vi "Write Master Motor Controller Config.vi"(8 "error in (no error)":errorcluster, 10 "Master Motor Controller Config":T1, 11 "Comp Motors with Encoders in":refnum<class "Comp Motors with Encoders.lvclass">) -> (0 "error out":errorcluster, 3 "Comp Motors with Encoders out":refnum<class "Comp Motors with Encoders.lvclass">)   [LabVIEW 2014, in "Comp Motors with Encoders.lvlib" / "Comp Motors with Encoders.lvclass"]
uses:
  Comp Motors with Encoders.lvclass
  Motor Controller Config.ctl
  Comp Motors with Encoders.lvclass/Comp Motors with Encoders.ctl
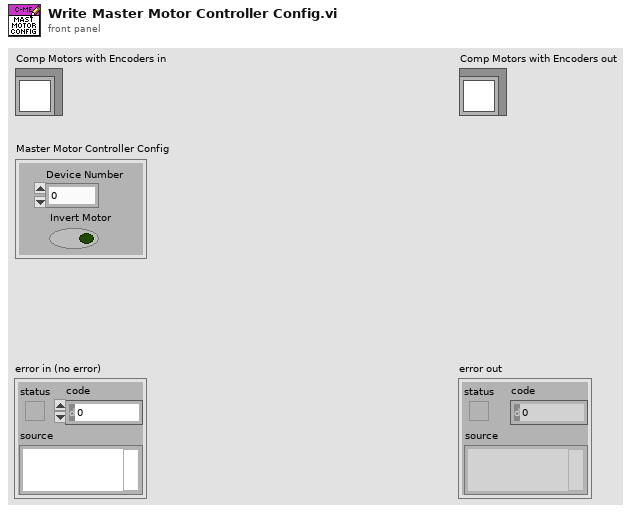
[diagram p1: front panel]
types:
  T1 = typedef "Comp Motors with Encoders.lvlib/Comp Motors with Encoders.lvclass/Motor Controller Config.ctl" = cluster{"Device Number":u8, "Invert Motor":bool}
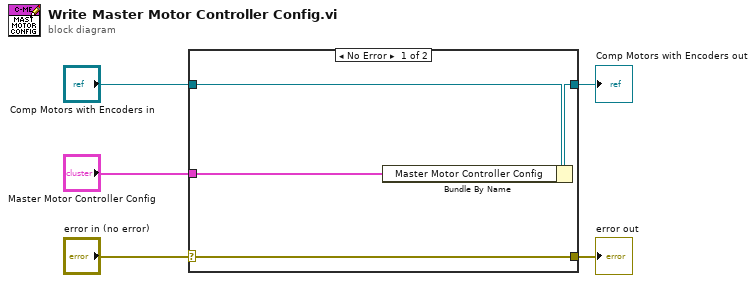
[diagram p0: block diagram]
diagram:
  n1 = case shown="No Error" "error in (no error)" {
    selector: "error in (no error)" -> [w9 w10]
    tunnel: [w9 w10] -> w4
    tunnel: [w7 w11] -> w2
    tunnel: "Comp Motors with Encoders in" -> [w8 w11]
    tunnel: "Master Motor Controller Config" -> [w6 _]
    frame No Error {
      n2 = Bundle By Name(cluster=w8, "Master Motor Controller Config"=w6) -> (w7:refnum<class "Comp Motors with Encoders.lvclass">)
    }
    frame Error {
    }
  }
  "error out" <- w4
  "Comp Motors with Encoders out" <- w2
